vi "SV Append Data (N Ch) (DBL).vi"(7 "reset (F)":bool, 10 "maximum length (-1 = unlimited)":i32=-1, 11 "data in":dbl[](array[numeric])) -> (3 "appended data":dbl[][](array[numeric]))   [LabVIEW 2017]
doc: "Use this VI to buffer data by appending input data to previously buffered data. Set the <B>maximum length</B> to set the buffered array size. The VI functions like a FIFO (First In, First Out) buffer, meaning that the oldest data is overwritten as new elements are added to the buffer. Wire data to the <B>data in</B> input to determine the polymorphic instance to use or manually select the instance."
panel:
  # "Ch"
  # "sample"
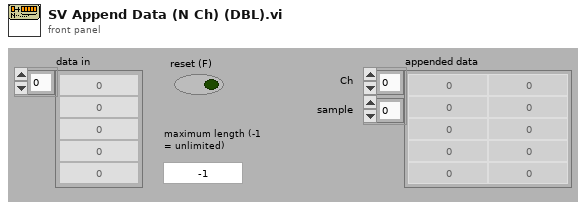
[diagram p1: front panel]
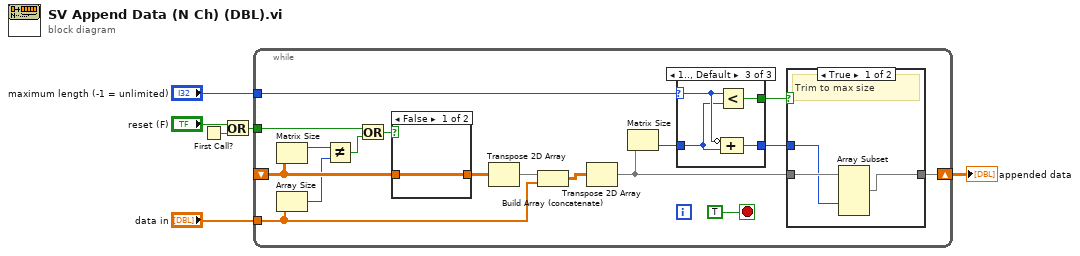
[diagram p0: block diagram]
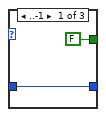
[diagram p2: hidden frame]
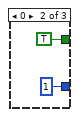
[diagram p3: hidden frame]
diagram:
  n1 = First Call?() -> (First Call?: T/F=w1:bool)
  n2 = Or(x="reset (F)", y=w1) -> (x .or. y?=w4:bool)
  n3 = while {
    tunnel: "data in" -> [w11]
    shift-right: [w8] -> w3
    shift-left: _ -> [w20]
    tunnel: "maximum length (-1 = unlimited)" -> [w21]
    tunnel: w4 -> [w16]
    stop <- TRUE stop-if-true
    n4 = Matrix Size(0:w20) -> (1:w19:i32)  [unwired: 1 out]
    n5 = Array Size(array=w11) -> (size(s)=w18:i32)
    n6 = Not Equal?(x=w19, y=w18) -> (x != y?=w17:bool)
    n7 = Or(x=w16, y=w17) -> (x .or. y?=w15:bool)
    n8 = case shown="False" w15 {
      tunnel: [w36 _] -> w13
      tunnel: w20 -> [w36 _]
      frame False {
      }
      frame True {
      }
    }
    n9 = Transpose 2D Array(2D array=w13) -> (transposed array=w12:dbl[][])
    n10 = Build Array (concatenate)(w12, w11) -> (w14:dbl[][])
    n11 = Transpose 2D Array(2D array=w14) -> (transposed array=w9:dbl[][])
    n12 = Matrix Size(0:w9) -> (2:w10:i32)  [unwired: 1 out]
    n13 = case shown="1.., Default" w21 {
      selector: w21 -> [_ _ w30]
      tunnel: [FALSE TRUE w31] -> w23
      tunnel: [w25 1 ("matrix") w29] -> w22
      tunnel: w10 -> [w25 _ w28]
      frame ..-1 {
      }
      frame 0 {
      }
      frame 1.., Default {
        n14 = Less?(x=w30, y=w28) -> (x < y?=w31:bool)
        n15 = Compound Arithmetic op=ADD(invert w30, w28) -> (w29:i32)
      }
    }
    n16 = case shown="True" w23 {
      tunnel: [w33 w35] -> w8
      tunnel: w22 -> [w32 _]
      tunnel: w9 -> [w34 w35]
      frame True {
        # "Trim to max size"
        n17 = Array Subset(array=w34, index (col)=w32) -> (w33:dbl[][])  [unwired: 3 in]
      }
      frame False {
        # "pass appended data"
      }
    }
  }
  "appended data" <- w3
